vi "Normalized_sound.vi"(11 "signal IN":dbl[](array[numeric])) -> (3 "signal OUT":dbl[](array[numeric]))   [LabVIEW 2022 SP3]
panel:
  out "Waveform Output":dbl[](graph)
  out "Waveform Input":dbl[](graph)
  out "Numeric":dbl
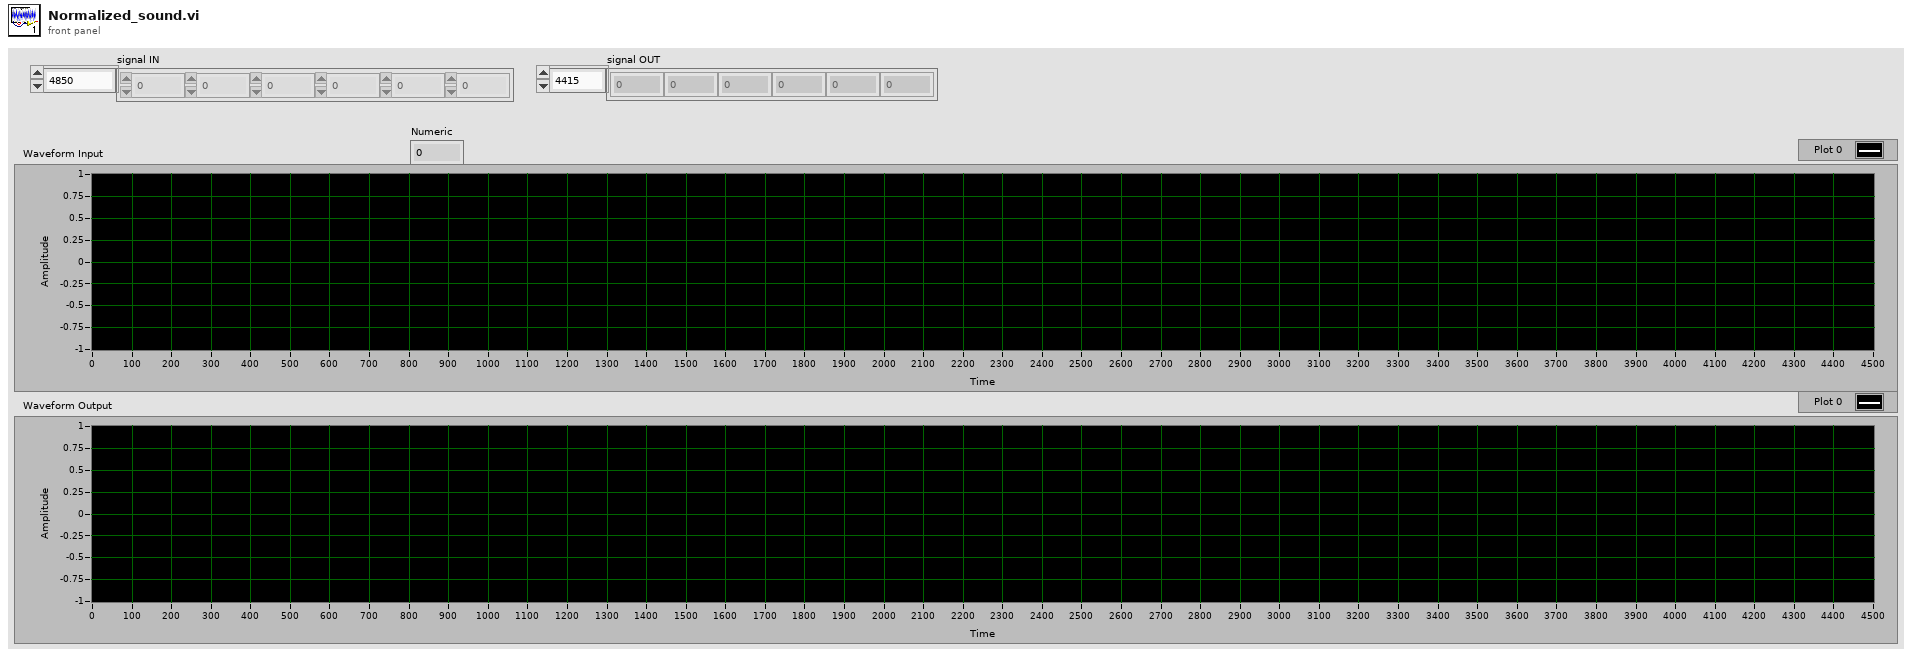
[diagram p1: front panel]
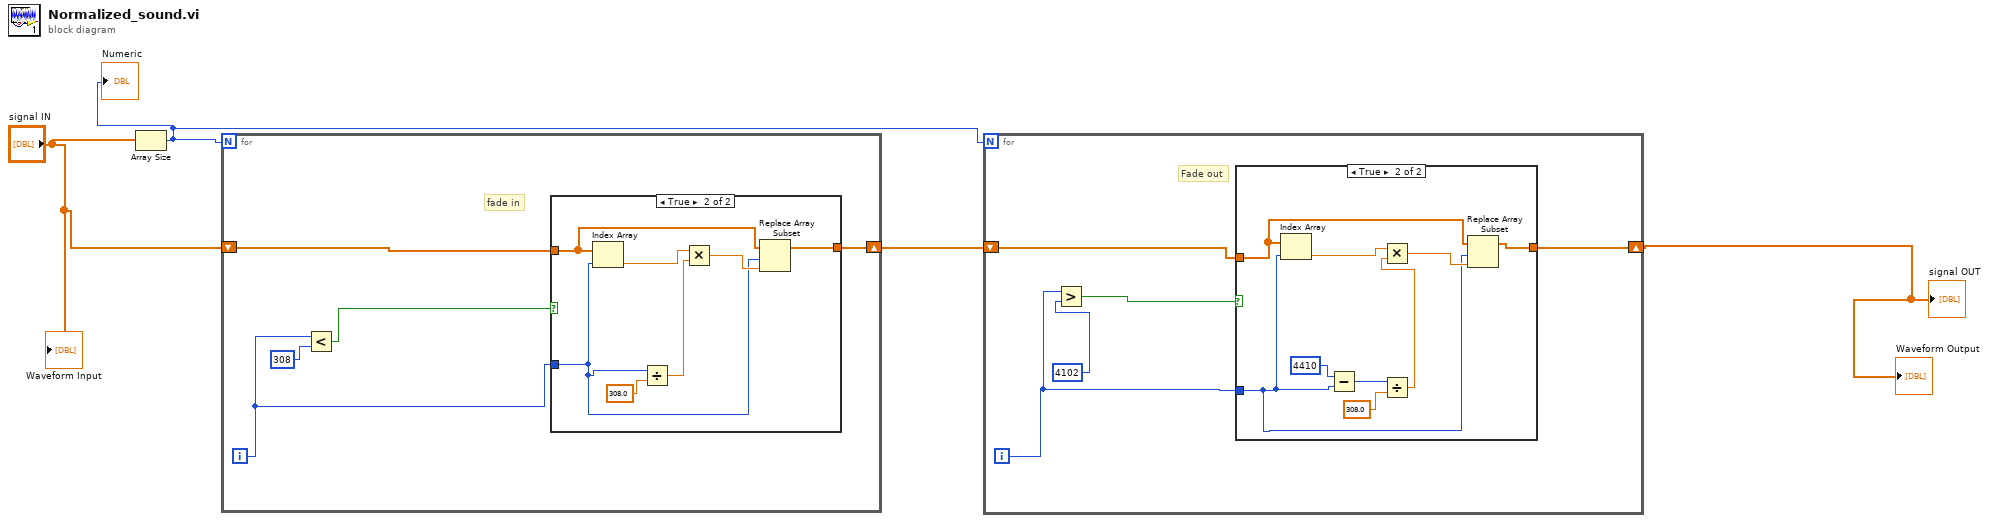
[diagram p0: block diagram]
diagram:
  n1 = Array Size(array="signal IN") -> (size(s)=w2:i32)
  "Numeric" <- w2
  n2 = for {
    N: w2 -> [_]
    shift-right: [w5] -> w4
    shift-left: "signal IN" -> [w8]
    i -> [w7]
    # "fade in"
    n3 = Less?(x=w7, y=308) -> (x < y?=w6:bool)
    n4 = case shown="True" w6 {
      tunnel: w8 -> [w10 w15]
      tunnel: w7 -> [_ w13]
      tunnel: [w10 w14] -> w5
      frame False {
      }
      frame True {
        n5 = Index Array(array=w15, index=w13) -> (element=w17:dbl)
        n6 = Divide(x=w13, y=308.0) -> (x/y=w11:dbl)
        n7 = Multiply(x=w17, y=w11) -> (x*y=w16:dbl)
        n8 = Replace Array Subset(array=w15, new element=w16, index=w13) -> (w14:dbl[])
      }
    }
  }
  n9 = for {
    N: w2 -> [_]
    shift-right: [w19] -> w1
    shift-left: w4 -> [w21]
    i -> [w20]
    # "Fade out"
    n10 = Greater?(x=w20, y=4102) -> (0:w18:bool)
    n11 = case shown="True" w18 {
      tunnel: w20 -> [_ w24]
      tunnel: w21 -> [w23 w28]
      tunnel: [w23 w26] -> w19
      frame False {
      }
      frame True {
        n12 = Index Array(array=w28, index=w24) -> (element=w29:dbl)
        n13 = Subtract(x=4410, y=w24) -> (x-y=w32:i32)
        n14 = Divide(x=w32, y=308.0) -> (x/y=w30:dbl)
        n15 = Multiply(x=w29, y=w30) -> (x*y=w27:dbl)
        n16 = Replace Array Subset(array=w28, new element=w27, index=w24) -> (w26:dbl[])
      }
    }
  }
  "signal OUT" <- w1
  "Waveform Output" <- w1
  "Waveform Input" <- "signal IN"
